vi "TextFit_Place String Line in Icon.vi"(4 "Frame":T1, 5 "Color Set":T2={"BG"=65793, "FG"=239}, 6 "Justify":T3, 7 "Starting Position":T6={"Left"=2, "Top"=6}, 8 "Error":errorcluster, 9 "Max Width":i32=30, 10 "String":string, 11 "ICON":T4 caption="Icon") -> (0 "Error Out":errorcluster, 1 "Fit Result Out":T5, 2 "Final Size Out":i32=30, 3 "ICON Out":T4)   [LabVIEW 2014]
doc: "Draws the String input in the icon at the starting position."
uses:
  Controls/String_Picture/Picture_Icon.ctl
  Controls/Cluster/Cluster_Top Left position.ctl
  Controls/Enum/ENUM RB_Fit Result.ctl
  Controls/Enum/ENUM_Text Justify.ctl
  Controls/Cluster/Cluster_Text Color Set.ctl
  Controls/Enum/ENUM_Frame Template Select.ctl
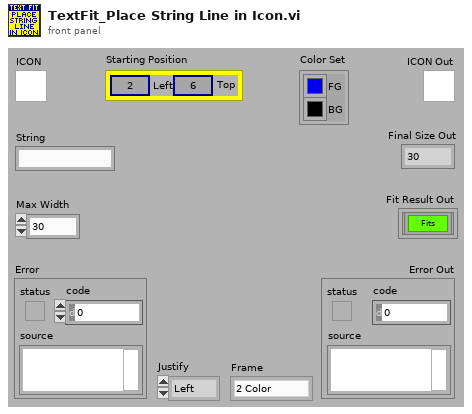
[diagram p1: front panel]
types:
  T1 = typedef "ENUM_Frame Template Select.ctl" = enum16{"2 Color", "5 Color"}
  T2 = typedef "Cluster_Text Color Set.ctl" = cluster{"BG":u32, "FG":u32}
  T3 = typedef "ENUM_Text Justify.ctl" = enum16{"Left", "Center", "Right"}
  T4 = typedef "Picture_Icon.ctl" = picture
  T5 = typedef "ENUM RB_Fit Result.ctl" = enum32{"Fits", "Almost Fits", "NO Fit"}
  T6 = typedef "Cluster_Top Left position.ctl" = cluster{"Left":i32, "Top":i32}
  T7 = typedef "Cluster_Character Size and Priority Data.ctl" = cluster{"Char":T8, "Font Size":T9, "Pixel width":i32, "Priority":i32, "Order":i32, "Index":i32}
  T8 = typedef "String Char Normal.ctl" = string
  T9 = typedef "ENUM_Font Size Select.ctl" = enum16{"Wide", "Med", "Thin"}
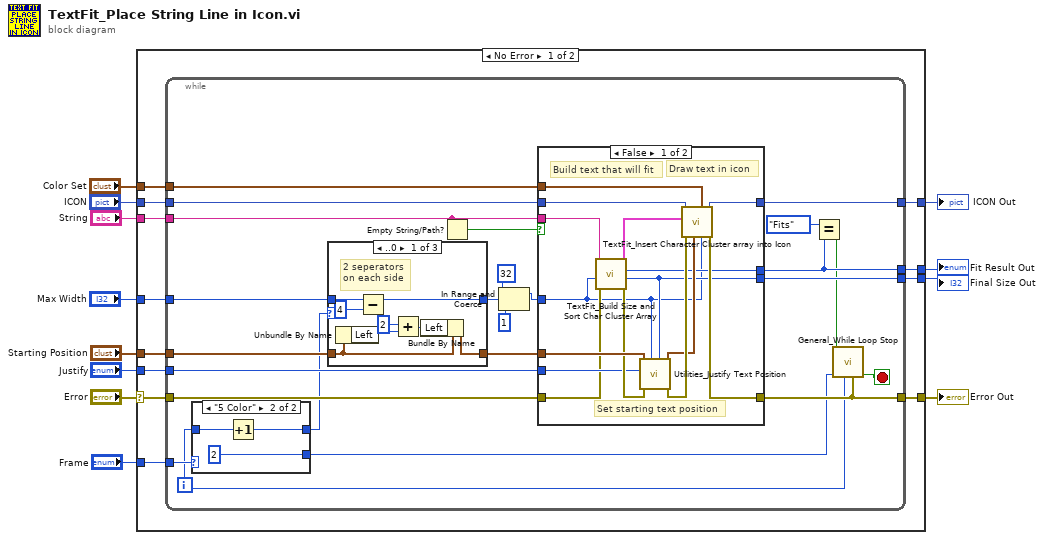
[diagram p0: block diagram]
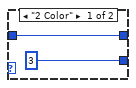
[diagram p2: hidden frame]
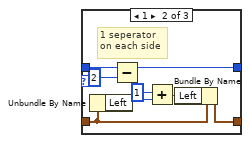
[diagram p3: hidden frame]
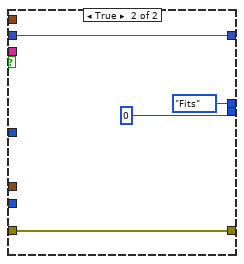
[diagram p5: hidden frame]
diagram:
  n1 = case shown="No Error" "Error" {
    selector: "Error" -> [w16 w91]
    tunnel: "ICON" -> [w24 w92]
    tunnel: [w23 w91] -> w11
    tunnel: [w22 w92] -> w10
    tunnel: "Starting Position" -> [w21 _]
    tunnel: [w20 _] -> w8
    tunnel: "Max Width" -> [w15 _]
    tunnel: [w19 _] -> w6
    tunnel: "Justify" -> [w18 _]
    tunnel: "Color Set" -> [w17 _]
    tunnel: "String" -> [w14 _]
    tunnel: "Frame" -> [w13 _]
    frame No Error {
      n2 = while {
        tunnel: w24 -> [w48]
        tunnel: [w40] -> w23
        tunnel: [w47] -> w22
        tunnel: w21 -> [w29]
        tunnel: [w39] -> w20
        tunnel: [w46] -> w19
        tunnel: w18 -> [w45]
        tunnel: w17 -> [w44]
        tunnel: w16 -> [w43]
        tunnel: w15 -> [w35]
        tunnel: w14 -> [w41]
        tunnel: w13 -> [w27]
        i -> [w26]
        stop <- w30 stop-if-true
        n3 = case shown="\"5 Color\"" w27 {
          tunnel: [3 ("Array Size In") 2 ("Array Size In")] -> w36
          tunnel: [w49 w51] -> w25
          tunnel: w26 -> [w49 w52]
          frame "2 Color" {
          }
          frame "5 Color" {
            n4 = Increment(x=w52) -> (x+1=w51:i32)
          }
        }
        n5 = case shown="..0" w25 {
          tunnel: w35 -> [w61 w69 w71]
          tunnel: [w59 w67 w71] -> w34
          tunnel: w29 -> [w55 w63 w70]
          tunnel: [w54 w62 w70] -> w28
          frame ..0 {
            # "2 seperators\non each side"
            n6 = Unbundle By Name(w55) -> ("Left"=w58:i32)
            n7 = Subtract(x=w61, y=4) -> (x-y=w59:i32)
            n8 = Add(x=2, y=w58) -> (x+y=w56:i32)
            n9 = Bundle By Name(cluster=w55, "Left"=w56) -> (w54:T6)
          }
          frame 1 {
            # "1 seperator\non each side"
            n10 = Unbundle By Name(w63) -> ("Left"=w66:i32)
            n11 = Subtract(x=w69, y=2) -> (x-y=w67:i32)
            n12 = Add(x=1, y=w66) -> (x+y=w64:i32)
            n13 = Bundle By Name(cluster=w63, "Left"=w64) -> (w62:T6)
          }
          frame 2.. {
            # "0 seperators"
          }
        }
        n14 = Empty String/Path?(string/path=w41) -> (empty?=w42:bool)
        n15 = In Range and Coerce(upper limit=32, x=w34, lower limit=1) -> (coerced(x)=w33:i32)  [unwired: 1 out]
        n16 = case shown="False" w42 {
          tunnel: w48 -> [w86 w90]
          tunnel: [w85 w89] -> w40
          tunnel: [w83 w90] -> w47
          tunnel: w28 -> [w82 _]
          tunnel: [w78 ENUM_RB_Fit_Result."Fits" ("Fit Result Out")] -> w39
          tunnel: [w77 0 ("Final Size Out")] -> w46
          tunnel: w45 -> [w76 _]
          tunnel: w44 -> [w75 _]
          tunnel: w41 -> [w74 _]
          tunnel: w43 -> [w73 w89]
          tunnel: w33 -> [w72 _]
          frame False {
            # "Set starting text position"
            # "Draw text in icon"
            # "Build text that will fit"
            n17 = call "TextFit_Build Size and Sort Char Cluster Array.vi"("Error"=w73, "Size To Fit"=w72, "String"=w74) -> ("Error Out"=w81:errorcluster, "Final Size Out"=w77:i32, "Fit Result Out"=w78:T5, "Build Array Out"=w84:T7[])  [unwired: 5 in]
            n18 = call "Utilities_Justify Text Position.vi"("Final Size"=w77, "Max Width"=w72, "Error"=w81, "Justify"=w76, "Postion"=w82) -> ("Error Out"=w80:errorcluster, "Position Out"=w79:T6)  [unwired: 5 in]
            n19 = call "TextFit_Insert Character Cluster array into Icon.vi"("Max Width"=w72, "Color Set"=w75, "Starting Posiition"=w79, "Error"=w80, "Character Array"=w84, "ICON"=w86) -> ("Error Out"=w85:errorcluster, "ICON Out"=w83:T4)  [unwired: 4 in]
          }
          frame True {
          }
        }
        n20 = Equal?(x=ENUM_RB_Fit_Result."Fits", y=w39) -> (x = y?=w37:bool)
        n21 = call "General_While Loop Stop.vi"("Error In"=w40, "Index In"=w26, "Array Size In"=w36, "Stop 1 In"=w37) -> ("Stop Out3"=w30:bool)  [unwired: 3 in, 3 out]
      }
    }
    frame Error {
    }
  }
  "Final Size Out" <- w6
  "Fit Result Out" <- w8
  "ICON Out" <- w10
  "Error Out" <- w11
